vi "Get Fit Results String.vi"(7 "Plot Name":string, 8 "error in (no error)":errorcluster, 9 "Fit Parameters Uncertainties Cluster":variant, 10 "Fit Model":T1, 11 "Fit Parameters Cluster":variant) -> (0 "error out":errorcluster, 3 "Fit Results String":string)   [LabVIEW 2019]
uses:
  Fit Models.ctl
  Gaussian Fit Results v2.ctl
  Lorentzian Fit Results v2.ctl
  Asymmetric Gaussian Fit Results v2.ctl
  Asymmetric Lorentzian Fit Results v2.ctl
  Gaussian-Lorentzian Fit Results v2.ctl
  Lorentzian-Gaussian Fit Results v2.ctl
  Two H-Connected Gaussians Fit Parameters.ctl
  Two T-Connected Gaussians Fit Parameters.ctl
  Two T-Connected Asymmetric Gaussians Fit Parameters.ctl
  Two H-Connected Asymmetric Gaussians Fit Parameters.ctl
  Single Exponential Fit Parameters v2.ctl
  Double Exponential Fit Parameters v2.ctl
  2D Gaussian ACF Fit Results.ctl
  2D Gaussian + Blinking ACF Fit Results.ctl
  2D Gaussian + Flow ACF Fit Results.ctl
  3D Gaussian ACF Fit Results.ctl
  3D Gaussian + Blinking ACF Fit Results.ctl
  2D Gaussian ACF & 2D Gaussian ACF + Flow Fit Results.ctl
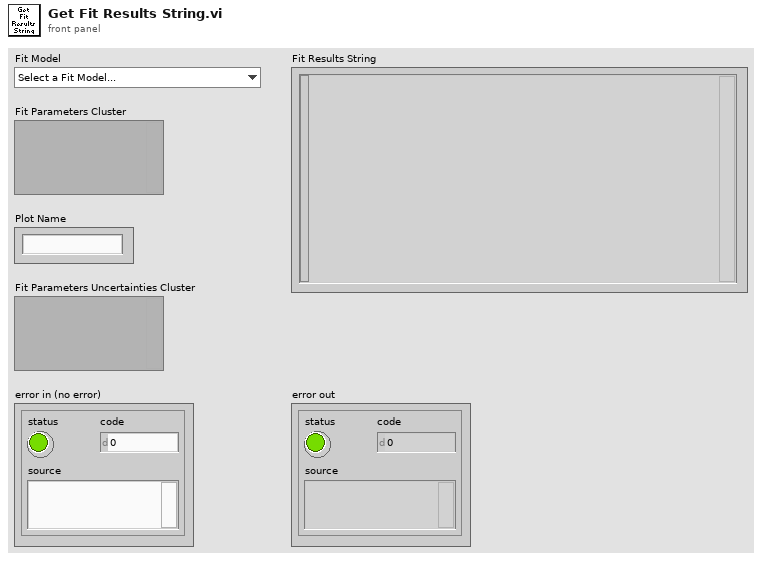
[diagram p1: front panel]
types:
  T1 = typedef "Fit Models.ctl" = enum16{"Select a Fit Model...", "           Single Peak", "Gaussian", "Asymmetric Gaussian", "Lorentzian", "Asymmetric Lorentzian", "Gaussian/Lorentzian", "Lorentzian/Gaussian", "           Double Peak", "Two Gaussians", "Two Asymmetric Gaussians", "Two H-Connected Gaussians", "Two T-Connected Gaussians", "Two H-Connected Asymmetric Gaussians", "Two T-Connected Asymmetric Gaussians", "           Triple Peak", "Three Gaussians", "Three Asymmetric Gaussians", "              Decays", "Single Exponential", "Two Exponentials", "               ACF", "2D Gaussian ACF", "2D Gaussian + Blinking ACF", "2D Gaussian + Flow ACF", "3D Gaussian ACF", "3D Gaussian + Blinking ACF", "             Multiplot", "2D Gaussian ACF & 2D Gaussian + Flow ACF"}
  T2 = typedef "Gaussian Fit Results v2.ctl" = cluster{"Amplitude":dbl, "Peak":dbl, "SDV":dbl, "FWHM":dbl, "Integral":dbl, "RMSE":dbl, "R^2":dbl}
  T3 = typedef "Lorentzian Fit Results v2.ctl" = cluster{"Amplitude":dbl, "Peak":dbl, "FWHM":dbl, "Integral":dbl, "RMSE":dbl, "R^2":dbl}
  T4 = typedef "Asymmetric Gaussian Fit Results v2.ctl" = cluster{"Amplitude":dbl, "Peak":dbl, "SDV-":dbl, "SDV+":dbl, "Mean":dbl, "SDV":dbl, "FWHM":dbl, "Integral":dbl, "RMSE":dbl, "R^2":dbl}
  T5 = typedef "Asymmetric Lorentzian Fit Results v2.ctl" = cluster{"Amplitude":dbl, "Peak":dbl, "FWHM-":dbl, "FWHM+":dbl, "Integral":dbl, "RMSE":dbl, "R^2":dbl}
  T6 = typedef "Gaussian-Lorentzian Fit Results v2.ctl" = cluster{"Amplitude":dbl, "Peak":dbl, "SDV-":dbl, "FWHM+":dbl, "Mean":dbl, "FWHM":dbl, "Integral":dbl, " RMSE":dbl, "R^2":dbl}
  T7 = typedef "Lorentzian-Gaussian Fit Results v2.ctl" = cluster{"Amplitude":dbl, "Peak":dbl, "FWHM-":dbl, "SDV+":dbl, "Mean":dbl, "FWHM":dbl, "Integral":dbl, "RMSE":dbl, "R^2":dbl}
  T8 = typedef "Two H-Connected Gaussians Fit Parameters.ctl" = cluster{"Gaussian Parameters":T2[], "Bridge Amplitude ":dbl}
  T9 = typedef "Two T-Connected Gaussians Fit Parameters.ctl" = cluster{"Gaussian Parameters":T2[], "Bridge Amplitude ":dbl, "Bridge Slope":dbl}
  T10 = typedef "Two T-Connected Asymmetric Gaussians Fit Parameters.ctl" = cluster{"Asymmetric Gaussian Parameters":T4[], "Bridge Amplitude":dbl, "Bridge Slope":dbl}
  T11 = typedef "Two H-Connected Asymmetric Gaussians Fit Parameters.ctl" = cluster{"Asymmetric Gaussian Parameters":T4[], "Bridge Amplitude":dbl}
  T12 = typedef "Single Exponential Fit Parameters v2.ctl" = cluster{"Amplitude":dbl, "Time Constant":dbl, "Mean":dbl, "SDV":dbl, "FWHM":dbl, "Integral":dbl, "MSE":dbl, "R^2":dbl}
  T13 = typedef "Double Exponential Fit Parameters v2.ctl" = cluster{"A1":dbl, "tau1":dbl, "A2":dbl, "tau2":dbl, "Mean":dbl, "SDV":dbl, "Integral":dbl, "MSE":dbl, "R^2":dbl}
  T14 = typedef "2D Gaussian ACF Fit Results.ctl" = cluster{"Amplitude":dbl, "Diffusion Time":dbl, "RMSE":dbl, "R^2":dbl}
  T15 = typedef "2D Gaussian + Blinking ACF Fit Results.ctl" = cluster{"Amplitude":dbl, "Diffusion Time":dbl, "Blinking Fraction":dbl, "Blinking Time Constant":dbl, "RMSE":dbl, "R^2":dbl}
  T16 = typedef "2D Gaussian + Flow ACF Fit Results.ctl" = cluster{"Amplitude":dbl, "Diffusion Time":dbl, "Translation Time":dbl, "RMSE":dbl, "R^2":dbl}
  T17 = typedef "3D Gaussian ACF Fit Results.ctl" = cluster{"Amplitude":dbl, "Diffusion Time":dbl, "Aspect Ratio":dbl, "RMSE":dbl, "R^2":dbl}
  T18 = typedef "3D Gaussian + Blinking ACF Fit Results.ctl" = cluster{"Amplitude":dbl, "Diffusion Time":dbl, "Aspect Ratio":dbl, "Blinking Fraction":dbl, "Blinking Time Constant":dbl, "RMSE":dbl, "R^2":dbl}
  T19 = typedef "2D Gaussian ACF & 2D Gaussian ACF + Flow Fit Results.ctl" = cluster{"Amplitude 1":dbl, "Diffusion Time":dbl, "Amplitude 2":dbl, "Translation Time":dbl, "RMSE":dbl, "R^2":dbl}
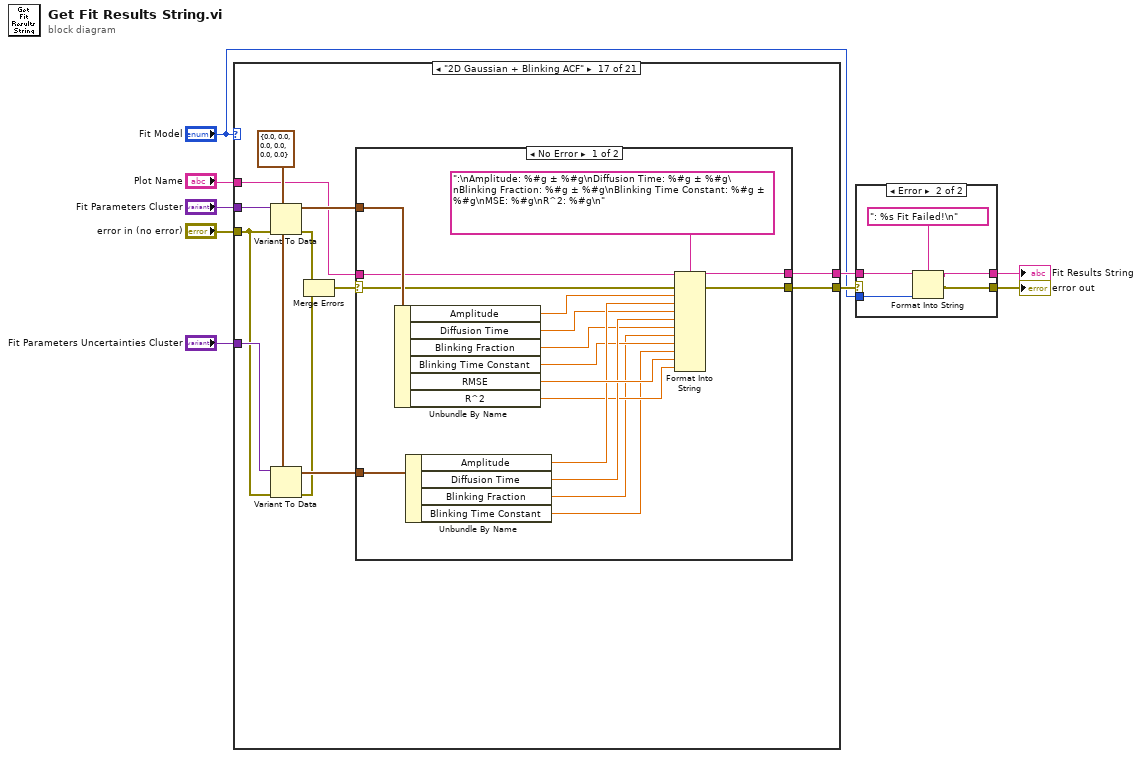
[diagram p0: block diagram]
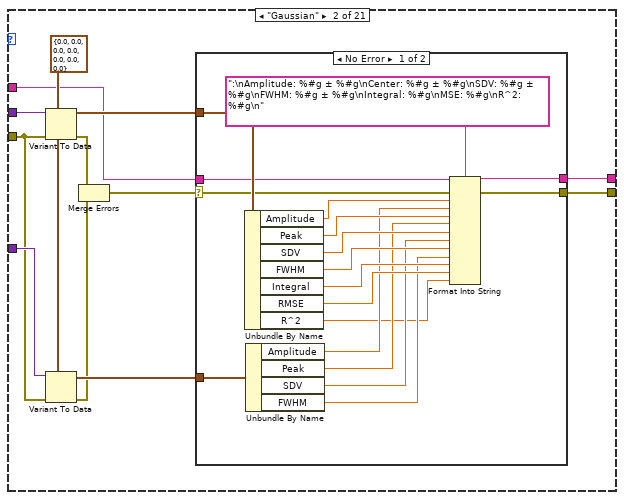
[diagram p4: hidden frame]
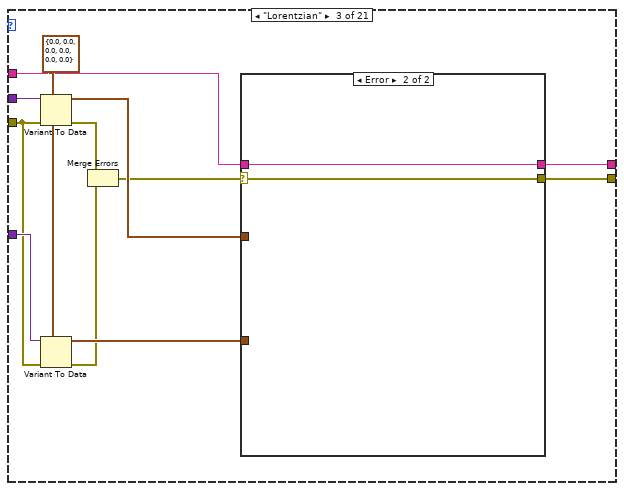
[diagram p6: hidden frame]
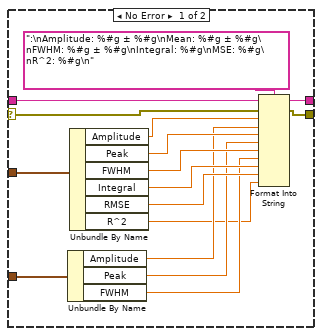
[diagram p7: hidden frame]
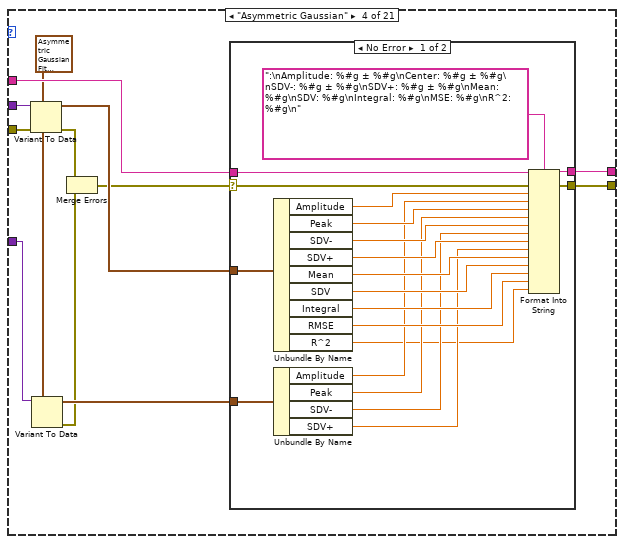
[diagram p8: hidden frame]
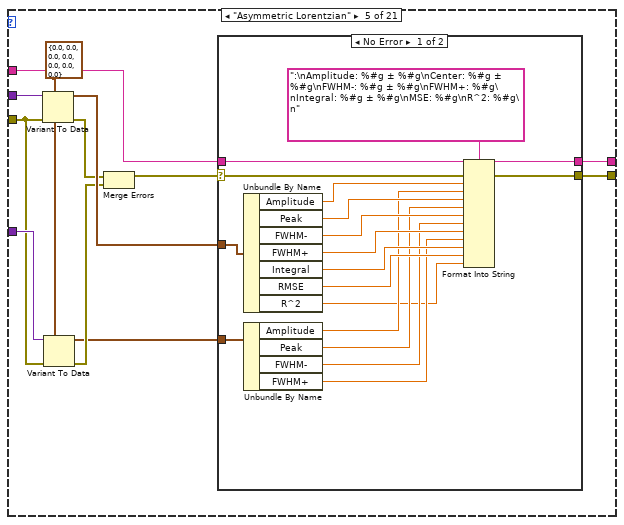
[diagram p10: hidden frame]
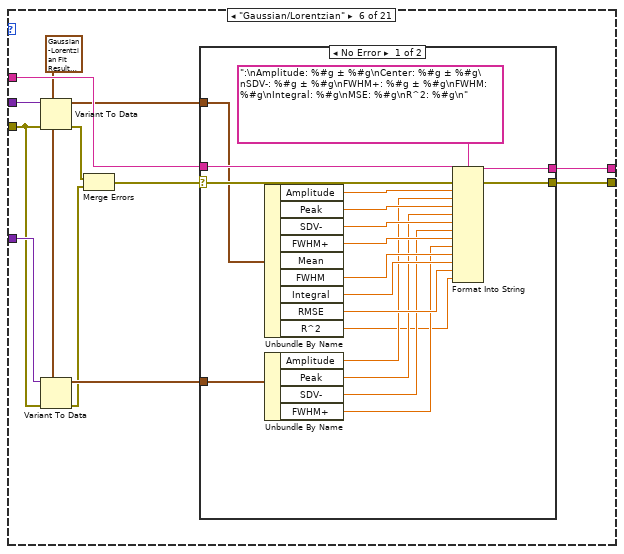
[diagram p12: hidden frame]
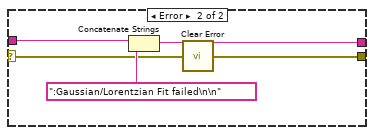
[diagram p13: hidden frame]
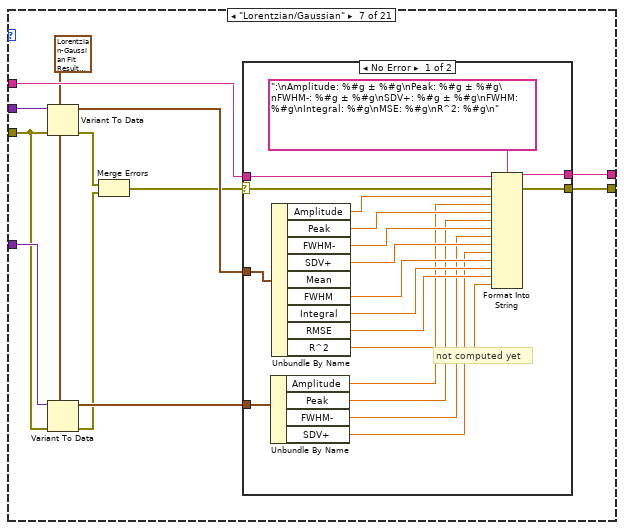
[diagram p14: hidden frame]
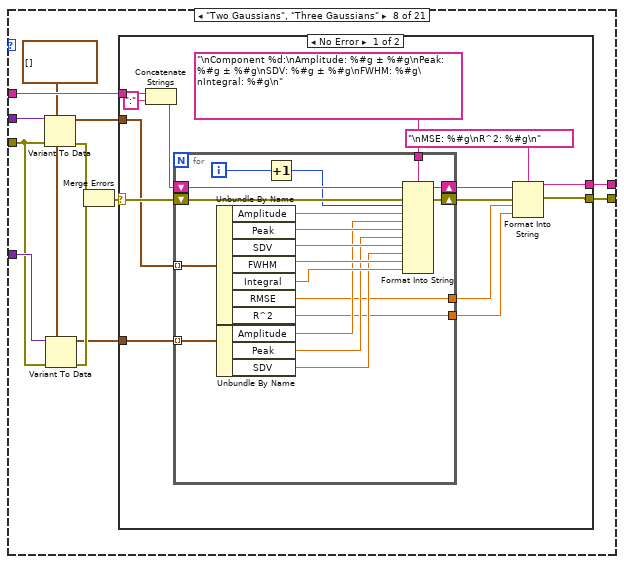
[diagram p16: hidden frame]
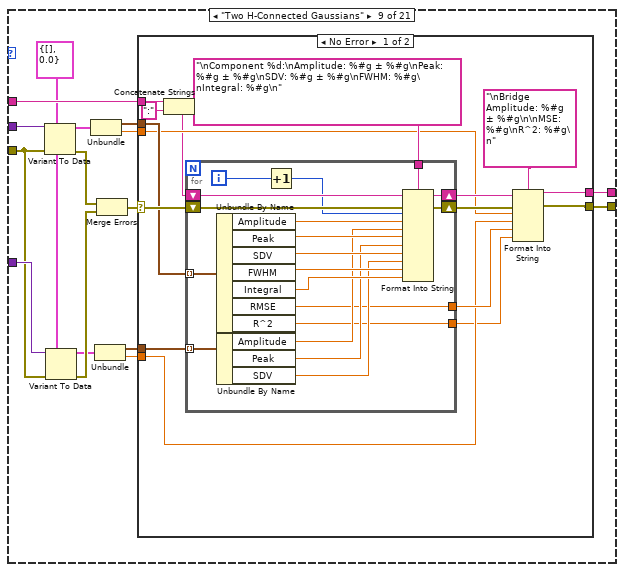
[diagram p18: hidden frame]
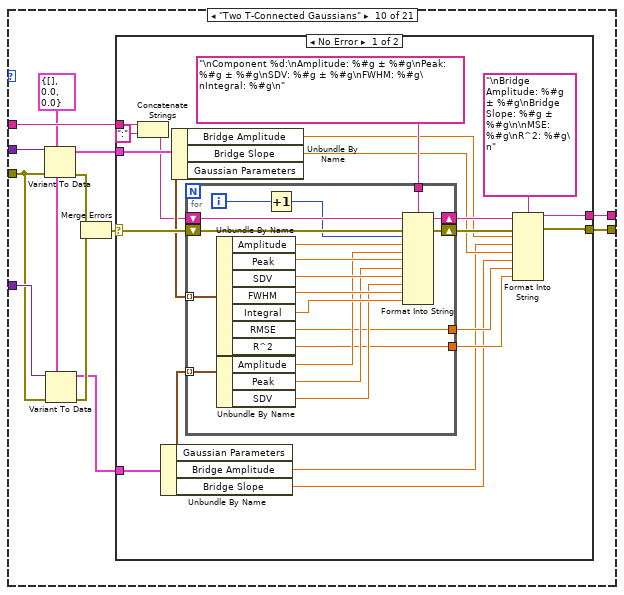
[diagram p20: hidden frame]
diagram:
  n1 = case shown="\"2D Gaussian + Blinking ACF\"" "Fit Model" {
    tunnel: "error in (no error)" -> [w10 w15 w46 w81 w110 w141 w175 w214 w265 w314 w366 w417 w474 w530 w561 w592 w619 w650 w679 w709 w742]
    tunnel: [w10 w22 w53 w83 w118 w149 w185 w218 w269 w318 w371 w422 w479 w533 w564 w599 w626 w657 w686 w715 w748] -> w5
    tunnel: [_ w21 w54 w84 w117 w150 w186 w219 w270 w319 w372 w423 w480 w534 w565 w598 w625 w656 w685 w714 w747] -> w3
    tunnel: "Fit Parameters Cluster" -> [_ w20 w52 w82 w115 w147 w183 w216 w267 w316 w369 w420 w477 w529 w563 w597 w624 w655 w684 w713 w746]
    tunnel: "Fit Parameters Uncertainties Cluster" -> [_ w18 w50 w76 w111 w142 w179 w215 w266 w315 w367 w418 w475 _ w562 w595 w622 w653 w682 w711 w744]
    tunnel: "Plot Name" -> [_ w11 w47 w80 w116 w148 w184 w217 w268 w317 w370 w421 w478 w524 w554 w588 w615 w646 w675 w705 w738]
    frame "Select a Fit Model...", Default {
    }
    frame "Gaussian" {
      w17 = T2 {"Amplitude"=0.0, "Peak"=0.0, "SDV"=0.0, "FWHM"=0.0, "Integral"=0.0, "RMSE"=0.0, "R^2"=0.0} ("Gaussian Fit Parameters")
      n2 = Variant To Data(error in=w15, type=w17, Variant=w20) -> (data=w19:T2, error out=w14:errorcluster)
      n3 = Variant To Data(error in=w15, type=w17, Variant=w18) -> (data=w16:T2, error out=w13:errorcluster)
      n4 = Merge Errors(w14, w13) -> (w12:errorcluster)
      n5 = case shown="No Error" w12 {
        selector: w12 -> [w30 w41]
        tunnel: [w40 w41] -> w22
        tunnel: [w39 w42] -> w21
        tunnel: w11 -> [w24 w42]
        tunnel: w19 -> [w37 _]
        tunnel: w16 -> [w29 _]
        frame No Error {
          n6 = Unbundle By Name(w37) -> ("Amplitude"=w36:dbl, "Peak"=w35:dbl, "SDV"=w34:dbl, "FWHM"=w32:dbl, "Integral"=w33:dbl, "RMSE"=w31:dbl, "R^2"=w23:dbl)
          n7 = Unbundle By Name(w29) -> ("Amplitude"=w28:dbl, "Peak"=w27:dbl, "SDV"=w26:dbl, "FWHM"=w25:dbl)
          n8 = Format Into String(format string=":\nAmplitude: %#g ± %#g\nCenter: %#g ± %#g\nSDV: %#g ± %#g\nFWHM: %#g ± %#g\nIntegral: %#g\nMSE: %#g\nR^2: %#g\n", initial string=w24, error in=w30, w36, w28, w35, w27, w34, w26, w32, w25, w33, w31, w23) -> (resulting string=w39:string, error out=w40:errorcluster)
        }
        frame Error {
        }
      }
    }
    frame "Lorentzian" {
      w48 = T3 {"Amplitude"=0.0, "Peak"=0.0, "FWHM"=0.0, "Integral"=0.0, "RMSE"=0.0, "R^2"=0.0} ("Lorentz Fit Parameters")
      n9 = Variant To Data(error in=w46, type=w48, Variant=w52) -> (data=w51:T3, error out=w45:errorcluster)
      n10 = Variant To Data(error in=w46, type=w48, Variant=w50) -> (data=w49:T3, error out=w44:errorcluster)
      n11 = Merge Errors(w45, w44) -> (w43:errorcluster)
      n12 = case shown="Error" w43 {
        selector: w43 -> [w61 w71]
        tunnel: w47 -> [w70 w72]
        tunnel: w51 -> [w69 _]
        tunnel: [w63 w72] -> w54
        tunnel: [w62 w71] -> w53
        tunnel: w49 -> [w59 _]
        frame No Error {
          n13 = Unbundle By Name(w59) -> ("Amplitude"=w58:dbl, "Peak"=w57:dbl, "FWHM"=w56:dbl)
          n14 = Unbundle By Name(w69) -> ("Amplitude"=w67:dbl, "Peak"=w68:dbl, "FWHM"=w66:dbl, "Integral"=w65:dbl, "RMSE"=w64:dbl, "R^2"=w55:dbl)
          n15 = Format Into String(format string=":\nAmplitude: %#g ± %#g\nMean: %#g ± %#g\nFWHM: %#g ± %#g\nIntegral: %#g\nMSE: %#g\nR^2: %#g\n", initial string=w70, error in=w61, w67, w58, w68, w57, w66, w56, w65, w64, w55) -> (resulting string=w63:string, error out=w62:errorcluster)
        }
        frame Error {
        }
      }
    }
    frame "Asymmetric Gaussian" {
      w78 = T4 {"Amplitude"=0.0, "Peak"=0.0, "SDV-"=0.0, "SDV+"=0.0, "Mean"=0.0, "SDV"=0.0, "FWHM"=0.0, "Integral"=0.0, "RMSE"=0.0, "R^2"=0.0} ("Asymmetric Gaussian Fit Parameters")
      n16 = Variant To Data(error in=w81, type=w78, Variant=w82) -> (data=w79:T4, error out=w75:errorcluster)
      n17 = Variant To Data(type=w78, Variant=w76) -> (data=w77:T4, error out=w74:errorcluster)  [unwired: 1 in]
      n18 = Merge Errors(w75, w74) -> (w73:errorcluster)
      n19 = case shown="No Error" w73 {
        selector: w73 -> [w102 w106]
        tunnel: w80 -> [w104 w105]
        tunnel: w79 -> [w91 _]
        tunnel: [w93 w105] -> w84
        tunnel: [w92 w106] -> w83
        tunnel: w77 -> [w90 _]
        frame No Error {
          n20 = Unbundle By Name(w91) -> ("Amplitude"=w98:dbl, "Peak"=w101:dbl, "SDV-"=w100:dbl, "SDV+"=w99:dbl, "Mean"=w97:dbl, "SDV"=w96:dbl, "Integral"=w95:dbl, "RMSE"=w94:dbl, "R^2"=w85:dbl)
          n21 = Unbundle By Name(w90) -> ("Amplitude"=w89:dbl, "Peak"=w88:dbl, "SDV-"=w87:dbl, "SDV+"=w86:dbl)
          n22 = Format Into String(format string=":\nAmplitude: %#g ± %#g\nCenter: %#g ± %#g\nSDV-: %#g ± %#g\nSDV+: %#g ± %#g\nMean: %#g\nSDV: %#g\nIntegral: %#g\nMSE: %#g\nR^2: %#g\n", initial string=w104, error in=w102, w98, w89, w101, w88, w100, w87, w99, w86, w97, w96, w95, w94, w85) -> (resulting string=w93:string, error out=w92:errorcluster)
        }
        frame Error {
        }
      }
    }
    frame "Asymmetric Lorentzian" {
      w112 = T5 {"Amplitude"=0.0, "Peak"=0.0, "FWHM-"=0.0, "FWHM+"=0.0, "Integral"=0.0, "RMSE"=0.0, "R^2"=0.0} ("Asymmetric Lorentz Fit Parameters")
      n23 = Variant To Data(error in=w110, type=w112, Variant=w115) -> (data=w114:T5, error out=w113:errorcluster)
      n24 = Variant To Data(error in=w110, type=w112, Variant=w111) -> (data=w108:T5, error out=w109:errorcluster)
      n25 = Merge Errors(w113, w109) -> (w107:errorcluster)
      n26 = case shown="No Error" w107 {
        selector: w107 -> [w135 w138]
        tunnel: [w128 w138] -> w118
        tunnel: [w127 w137] -> w117
        tunnel: w116 -> [w122 w137]
        tunnel: w114 -> [w121 _]
        tunnel: w108 -> [w120 _]
        frame No Error {
          n27 = Unbundle By Name(w121) -> ("Amplitude"=w131:dbl, "Peak"=w134:dbl, "FWHM-"=w133:dbl, "FWHM+"=w132:dbl, "Integral"=w130:dbl, "RMSE"=w129:dbl, "R^2"=w119:dbl)
          n28 = Unbundle By Name(w120) -> ("Amplitude"=w126:dbl, "Peak"=w125:dbl, "FWHM-"=w124:dbl, "FWHM+"=w123:dbl)
          n29 = Format Into String(format string=":\nAmplitude: %#g ± %#g\nCenter: %#g ± %#g\nFWHM-: %#g ± %#g\nFWHM+: %#g\nIntegral: %#g ± %#g\nMSE: %#g\nR^2: %#g\n", initial string=w122, error in=w135, w131, w126, w134, w125, w133, w124, w132, w123, w130, w129, w119) -> (resulting string=w127:string, error out=w128:errorcluster)
        }
        frame Error {
        }
      }
    }
    frame "Gaussian/Lorentzian" {
      w143 = T6 {"Amplitude"=0.0, "Peak"=0.0, "SDV-"=0.0, "FWHM+"=0.0, "Mean"=0.0, "FWHM"=0.0, "Integral"=0.0, " RMSE"=0.0, "R^2"=0.0} ("Gaussian/Lorentzian Fit Parameters")
      n30 = Variant To Data(error in=w141, type=w143, Variant=w147) -> (data=w144:T6, error out=w146:errorcluster)
      n31 = Variant To Data(error in=w141, type=w143, Variant=w142) -> (data=w140:T6, error out=w139:errorcluster)
      n32 = Merge Errors(w146, w139) -> (w145:errorcluster)
      n33 = case shown="No Error" w145 {
        selector: w145 -> [w167 w171]
        tunnel: w148 -> [w169 w173]
        tunnel: [w159 w172] -> w150
        tunnel: [w158 w170] -> w149
        tunnel: w144 -> [w153 _]
        tunnel: w140 -> [w152 _]
        frame No Error {
          n34 = Unbundle By Name(w153) -> ("Amplitude"=w165:dbl, "Peak"=w166:dbl, "SDV-"=w164:dbl, "FWHM+"=w163:dbl, "FWHM"=w162:dbl, "Integral"=w161:dbl, "RMSE"=w160:dbl, "R^2"=w151:dbl)  [unwired: 1 out]
          n35 = Unbundle By Name(w152) -> ("Amplitude"=w157:dbl, "Peak"=w156:dbl, "SDV-"=w155:dbl, "FWHM+"=w154:dbl)
          n36 = Format Into String(format string=":\nAmplitude: %#g ± %#g\nCenter: %#g ± %#g\nSDV-: %#g ± %#g\nFWHM+: %#g ± %#g\nFWHM: %#g\nIntegral: %#g\nMSE: %#g\nR^2: %#g\n", initial string=w169, error in=w167, w165, w157, w166, w156, w164, w155, w163, w154, w162, w161, w160, w151) -> (resulting string=w159:string, error out=w158:errorcluster)
        }
        frame Error {
          n37 = Concatenate Strings(w173, ":Gaussian/Lorentzian Fit failed\n\n" ("format string")) -> (w172:string)
          n38 = call "Clear Error.vi"("Error In"=w171) -> ("no Error Out"=w170:errorcluster)  [unwired: 8 in]
        }
      }
    }
    frame "Lorentzian/Gaussian" {
      w178 = T7 {"Amplitude"=0.0, "Peak"=0.0, "FWHM-"=0.0, "SDV+"=0.0, "Mean"=0.0, "FWHM"=0.0, "Integral"=0.0, "RMSE"=0.0, "R^2"=0.0} ("Lorentzian/Gaussian Fit Parameters")
      n39 = Variant To Data(error in=w175, type=w178, Variant=w183) -> (data=w182:T7, error out=w181:errorcluster)
      n40 = Variant To Data(error in=w175, type=w178, Variant=w179) -> (data=w177:T7, error out=w176:errorcluster)
      n41 = Merge Errors(w181, w176) -> (w180:errorcluster)
      n42 = case shown="No Error" w180 {
        selector: w180 -> [w204 w207]
        tunnel: [w196 w206] -> w186
        tunnel: [w195 w207] -> w185
        tunnel: w184 -> [w190 w206]
        tunnel: w182 -> [w189 _]
        tunnel: w177 -> [w188 _]
        frame No Error {
          # "not computed yet"
          n43 = Unbundle By Name(w188) -> ("Amplitude"=w194:dbl, "Peak"=w193:dbl, "FWHM-"=w192:dbl, "SDV+"=w191:dbl)
          n44 = Unbundle By Name(w189) -> ("Amplitude"=w202:dbl, "Peak"=w203:dbl, "FWHM-"=w200:dbl, "SDV+"=w201:dbl, "FWHM"=w199:dbl, "Integral"=w198:dbl, "RMSE"=w197:dbl, "R^2"=w187:dbl)  [unwired: 1 out]
          n45 = Format Into String(format string=":\nAmplitude: %#g ± %#g\nPeak: %#g ± %#g\nFWHM-: %#g ± %#g\nSDV+: %#g ± %#g\nFWHM: %#g\nIntegral: %#g\nMSE: %#g\nR^2: %#g\n", initial string=w190, error in=w204, w202, w194, w203, w193, w200, w192, w201, w191, w199, w198, w197, w187) -> (resulting string=w196:string, error out=w195:errorcluster)
        }
        frame Error {
        }
      }
    }
    frame "Two Gaussians", "Three Gaussians" {
      w208 = T2[] [] ("Array")
      n46 = Variant To Data(error in=w214, type=w208, Variant=w216) -> (data=w210:T2[], error out=w213:errorcluster)
      n47 = Variant To Data(error in=w214, type=w208, Variant=w215) -> (data=w209:T2[], error out=w212:errorcluster)
      n48 = Merge Errors(w213, w212) -> (w211:errorcluster)
      n49 = case shown="No Error" w211 {
        selector: w211 -> [w232 w254]
        tunnel: [w227 w253] -> w219
        tunnel: [w225 w254] -> w218
        tunnel: w217 -> [w230 w253]
        tunnel: w210 -> [w229 _]
        tunnel: w209 -> [w228 _]
        frame No Error {
          n50 = Concatenate Strings(w230, ":" ("string")) -> (w221:string)
          n51 = for {
            tunnel: "\nComponent %d:\nAmplitude: %#g ± %#g\nPeak: %#g ± %#g\nSDV: %#g ± %#g\nFWHM: %#g\nIntegral: %#g\n" ("format string") -> [w252]
            shift-right: [w245] -> w226
            shift-left: w232 -> [w251]
            shift-right: [w246] -> w231
            shift-left: w221 -> [w244]
            tunnel: w229 -> [w237] mode=indexing
            tunnel: w228 -> [w236] mode=indexing
            tunnel: [w235] -> w223
            tunnel: [w234] -> w222
            i -> [w239]
            n52 = Unbundle By Name(w237) -> ("Amplitude"=w240:dbl, "Peak"=w250:dbl, "SDV"=w249:dbl, "FWHM"=w248:dbl, "Integral"=w247:dbl, "RMSE"=w235:dbl, "R^2"=w234:dbl)
            n53 = Unbundle By Name(w236) -> ("Amplitude"=w243:dbl, "Peak"=w242:dbl, "SDV"=w241:dbl)
            n54 = Increment(x=w239) -> (x+1=w238:i32)
            n55 = Format Into String(format string=w252, initial string=w244, error in=w251, w238, w240, w243, w250, w242, w249, w241, w248, w247) -> (resulting string=w246:string, error out=w245:errorcluster)
          }
          n56 = Format Into String(format string="\nMSE: %#g\nR^2: %#g\n", initial string=w231, error in=w226, w223, w222) -> (resulting string=w227:string, error out=w225:errorcluster)
        }
        frame Error {
        }
      }
    }
    frame "Two H-Connected Gaussians" {
      w259 = T8 {"Gaussian Parameters"=[], "Bridge Amplitude "=0.0} ("Bridged Gaussians Parameters")
      n57 = Variant To Data(error in=w265, type=w259, Variant=w267) -> (data=w261:T8, error out=w264:errorcluster)
      n58 = Variant To Data(error in=w265, type=w259, Variant=w266) -> (data=w260:T8, error out=w263:errorcluster)
      n59 = Unbundle(w261) -> ("Gaussian Parameters"=w258:T2[], "Bridge Amplitude"=w256:dbl)
      n60 = Unbundle(w260) -> ("Gaussian Parameters"=w257:T2[], "Bridge Amplitude"=w255:dbl)
      n61 = Merge Errors(w264, w263) -> (w262:errorcluster)
      n62 = case shown="No Error" w262 {
        selector: w262 -> [w285 w307]
        tunnel: [w281 w306] -> w270
        tunnel: [w279 w307] -> w269
        tunnel: w268 -> [w272 w306]
        tunnel: w258 -> [w283 _]
        tunnel: w257 -> [w282 _]
        tunnel: w256 -> [w275 _]
        tunnel: w255 -> [w276 _]
        frame No Error {
          n63 = Concatenate Strings(w272, ":" ("string")) -> (w271:string)
          n64 = for {
            tunnel: "\nComponent %d:\nAmplitude: %#g ± %#g\nPeak: %#g ± %#g\nSDV: %#g ± %#g\nFWHM: %#g\nIntegral: %#g\n" ("format string") -> [w305]
            shift-right: [w298] -> w280
            shift-left: w285 -> [w304]
            shift-right: [w299] -> w284
            shift-left: w271 -> [w297]
            tunnel: w283 -> [w290] mode=indexing
            tunnel: w282 -> [w289] mode=indexing
            tunnel: [w288] -> w277
            tunnel: [w287] -> w274
            i -> [w292]
            n65 = Unbundle By Name(w290) -> ("Amplitude"=w293:dbl, "Peak"=w303:dbl, "SDV"=w302:dbl, "FWHM"=w301:dbl, "Integral"=w300:dbl, "RMSE"=w288:dbl, "R^2"=w287:dbl)
            n66 = Unbundle By Name(w289) -> ("Amplitude"=w296:dbl, "Peak"=w295:dbl, "SDV"=w294:dbl)
            n67 = Increment(x=w292) -> (x+1=w291:i32)
            n68 = Format Into String(format string=w305, initial string=w297, error in=w304, w291, w293, w296, w303, w295, w302, w294, w301, w300) -> (resulting string=w299:string, error out=w298:errorcluster)
          }
          n69 = Format Into String(format string="\nBridge Amplitude: %#g ± %#g\n\nMSE: %#g\nR^2: %#g\n", initial string=w284, error in=w280, w275, w276, w277, w274) -> (resulting string=w281:string, error out=w279:errorcluster)
        }
        frame Error {
        }
      }
    }
    frame "Two T-Connected Gaussians" {
      w310 = T9 {"Gaussian Parameters"=[], "Bridge Amplitude "=0.0, "Bridge Slope"=0.0} ("Bridged Gaussians Parameters")
      n70 = Variant To Data(error in=w314, type=w310, Variant=w316) -> (data=w309:T9, error out=w313:errorcluster)
      n71 = Variant To Data(error in=w314, type=w310, Variant=w315) -> (data=w308:T9, error out=w312:errorcluster)
      n72 = Merge Errors(w313, w312) -> (w311:errorcluster)
      n73 = case shown="No Error" w311 {
        selector: w311 -> [w338 w360]
        tunnel: [w336 w359] -> w319
        tunnel: [w334 w360] -> w318
        tunnel: w317 -> [w321 w359]
        tunnel: w309 -> [w330 _]
        tunnel: w308 -> [w326 _]
        frame No Error {
          n74 = Concatenate Strings(w321, ":" ("string")) -> (w320:string)
          n75 = Unbundle By Name(w326) -> ("Gaussian Parameters"=w325:T2[], "Bridge Amplitude"=w324:dbl, "Bridge Slope"=w323:dbl)
          n76 = Unbundle By Name(w330) -> ("Bridge Amplitude"=w328:dbl, "Bridge Slope"=w327:dbl, "Gaussian Parameters"=w329:T2[])
          n77 = for {
            tunnel: "\nComponent %d:\nAmplitude: %#g ± %#g\nPeak: %#g ± %#g\nSDV: %#g ± %#g\nFWHM: %#g\nIntegral: %#g\n" ("format string") -> [w358]
            shift-right: [w351] -> w335
            shift-left: w338 -> [w357]
            shift-right: [w352] -> w337
            shift-left: w320 -> [w350]
            tunnel: w329 -> [w343] mode=indexing
            tunnel: w325 -> [w342] mode=indexing
            tunnel: [w341] -> w332
            tunnel: [w340] -> w331
            i -> [w345]
            n78 = Unbundle By Name(w343) -> ("Amplitude"=w346:dbl, "Peak"=w356:dbl, "SDV"=w355:dbl, "FWHM"=w354:dbl, "Integral"=w353:dbl, "RMSE"=w341:dbl, "R^2"=w340:dbl)
            n79 = Unbundle By Name(w342) -> ("Amplitude"=w349:dbl, "Peak"=w348:dbl, "SDV"=w347:dbl)
            n80 = Increment(x=w345) -> (x+1=w344:i32)
            n81 = Format Into String(format string=w358, initial string=w350, error in=w357, w344, w346, w349, w356, w348, w355, w347, w354, w353) -> (resulting string=w352:string, error out=w351:errorcluster)
          }
          n82 = Format Into String(format string="\nBridge Amplitude: %#g ± %#g\nBridge Slope: %#g ± %#g\n\nMSE: %#g\nR^2: %#g\n", initial string=w337, error in=w335, w328, w324, w327, w323, w332, w331) -> (resulting string=w336:string, error out=w334:errorcluster)
        }
        frame Error {
        }
      }
    }
    frame "Two Asymmetric Gaussians", "Three Asymmetric Gaussians" {
      w365 = T4[] [] ("Array")
      n83 = Variant To Data(error in=w366, type=w365, Variant=w367) -> (data=w361:T4[], error out=w364:errorcluster)
      n84 = Variant To Data(error in=w366, type=w365, Variant=w369) -> (data=w362:T4[], error out=w368:errorcluster)
      n85 = Merge Errors(w368, w364) -> (w363:errorcluster)
      n86 = case shown="No Error" w363 {
        selector: w363 -> [w385 w410]
        tunnel: w370 -> [w386 w411]
        tunnel: [w378 w411] -> w372
        tunnel: [w376 w410] -> w371
        tunnel: w362 -> [w384 _]
        tunnel: w361 -> [w383 _]
        frame No Error {
          n87 = Concatenate Strings(w386, ":" ("string")) -> (w381:string)
          n88 = for {
            shift-right: [w399] -> w379
            shift-left: w381 -> [w402]
            shift-right: [w400] -> w377
            shift-left: w385 -> [w401]
            tunnel: w384 -> [w398] mode=indexing
            tunnel: w383 -> [w397] mode=indexing
            tunnel: "\nComponent %d:\nAmplitude: %#g ± %#g\nCenter: %#g ± %#g\nSDV-: %#g ± %#g\nSDV+: %#g ± %#g\nMean: %#g\nSDV: %#g\nFWHM: %#g\nIntegral: %#g\n" ("format string") -> [w396]
            tunnel: [w388] -> w375
            tunnel: [w387] -> w373
            i -> [w394]
            n89 = Unbundle By Name(w398) -> ("Amplitude"=w395:dbl, "Peak"=w409:dbl, "SDV-"=w408:dbl, "SDV+"=w407:dbl, "Mean"=w406:dbl, "SDV"=w405:dbl, "FWHM"=w404:dbl, "Integral"=w403:dbl, "RMSE"=w388:dbl, "R^2"=w387:dbl)
            n90 = Unbundle By Name(w397) -> ("Amplitude"=w392:dbl, "Peak"=w391:dbl, "SDV-"=w390:dbl, "SDV+"=w389:dbl)
            n91 = Increment(x=w394) -> (x+1=w393:i32)
            n92 = Format Into String(format string=w396, initial string=w402, error in=w401, w393, w395, w392, w409, w391, w408, w390, w407, w389, w406, w405, w404, w403) -> (resulting string=w399:string, error out=w400:errorcluster)
          }
          n93 = Format Into String(format string="\nMSE: %#g\nR^2: %#g\n", initial string=w379, error in=w377, w375, w373) -> (resulting string=w378:string, error out=w376:errorcluster)
        }
        frame Error {
        }
      }
    }
    frame "Two T-Connected Asymmetric Gaussians" {
      w412 = T10 {"Asymmetric Gaussian Parameters"=[], "Bridge Amplitude"=0.0, "Bridge Slope"=0.0} ("Two T-Connected Asymmetric Gaussian Parameters")
      n94 = Variant To Data(error in=w417, type=w412, Variant=w418) -> (data=w413:T10, error out=w416:errorcluster)
      n95 = Variant To Data(error in=w417, type=w412, Variant=w420) -> (data=w414:T10, error out=w419:errorcluster)
      n96 = Merge Errors(w419, w416) -> (w415:errorcluster)
      n97 = case shown="No Error" w415 {
        selector: w415 -> [w442 w467]
        tunnel: w421 -> [w443 w468]
        tunnel: [w436 w468] -> w423
        tunnel: [w435 w467] -> w422
        tunnel: w414 -> [w441 _]
        tunnel: w413 -> [w427 _]
        frame No Error {
          n98 = Unbundle By Name(w441) -> ("Bridge Amplitude"=w431:dbl, "Bridge Slope"=w430:dbl, "Asymmetric Gaussian Parameters"=w428:T4[])
          n99 = Concatenate Strings(w443, ":" ("string")) -> (w439:string)
          n100 = Unbundle By Name(w427) -> ("Asymmetric Gaussian Parameters"=w426:T4[], "Bridge Amplitude"=w425:dbl, "Bridge Slope"=w424:dbl)
          n101 = for {
            shift-right: [w456] -> w437
            shift-left: w439 -> [w459]
            shift-right: [w457] -> w434
            shift-left: w442 -> [w458]
            tunnel: w428 -> [w455] mode=indexing
            tunnel: w426 -> [w454] mode=indexing
            tunnel: "\nComponent %d:\nAmplitude: %#g ± %#g\nCenter: %#g ± %#g\nSDV-: %#g ± %#g\nSDV+: %#g ± %#g\nMean: %#g\nSDV: %#g\nFWHM: %#g\nIntegral: %#g\n" ("format string") -> [w453]
            tunnel: [w445] -> w432
            tunnel: [w444] -> w429
            i -> [w451]
            n102 = Unbundle By Name(w455) -> ("Amplitude"=w452:dbl, "Peak"=w466:dbl, "SDV-"=w465:dbl, "SDV+"=w464:dbl, "Mean"=w463:dbl, "SDV"=w462:dbl, "FWHM"=w461:dbl, "Integral"=w460:dbl, "RMSE"=w445:dbl, "R^2"=w444:dbl)
            n103 = Unbundle By Name(w454) -> ("Amplitude"=w449:dbl, "Peak"=w448:dbl, "SDV-"=w447:dbl, "SDV+"=w446:dbl)
            n104 = Increment(x=w451) -> (x+1=w450:i32)
            n105 = Format Into String(format string=w453, initial string=w459, error in=w458, w450, w452, w449, w466, w448, w465, w447, w464, w446, w463, w462, w461, w460) -> (resulting string=w456:string, error out=w457:errorcluster)
          }
          n106 = Format Into String(format string="\nBridge Amplitude: %#g ± %#g\nBridge Slope: %#g ± %#g\n\nMSE: %#g\nR^2: %#g\n", initial string=w437, error in=w434, w431, w425, w430, w424, w432, w429) -> (resulting string=w436:string, error out=w435:errorcluster)
        }
        frame Error {
        }
      }
    }
    frame "Two H-Connected Asymmetric Gaussians" {
      w471 = T11 {"Asymmetric Gaussian Parameters"=[], "Bridge Amplitude"=0.0} ("output cluster")
      n107 = Variant To Data(error in=w474, type=w471, Variant=w475) -> (data=w469:T11, error out=w473:errorcluster)
      n108 = Variant To Data(error in=w474, type=w471, Variant=w477) -> (data=w470:T11, error out=w476:errorcluster)
      n109 = Merge Errors(w476, w473) -> (w472:errorcluster)
      n110 = case shown="No Error" w472 {
        selector: w472 -> [w497 w522]
        tunnel: w478 -> [w498 w523]
        tunnel: [w492 w523] -> w480
        tunnel: [w490 w522] -> w479
        tunnel: w470 -> [w485 _]
        tunnel: w469 -> [w484 _]
        frame No Error {
          n111 = Unbundle(w484) -> ("Asymmetric Gaussian Parameters"=w483:T4[], "Bridge Amplitude"=w482:dbl)
          n112 = Unbundle(w485) -> ("Asymmetric Gaussian Parameters"=w487:T4[], "Bridge Amplitude"=w486:dbl)
          n113 = Concatenate Strings(w498, ":" ("string")) -> (w495:string)
          n114 = for {
            shift-right: [w511] -> w493
            shift-left: w495 -> [w514]
            shift-right: [w512] -> w491
            shift-left: w497 -> [w513]
            tunnel: w487 -> [w510] mode=indexing
            tunnel: w483 -> [w509] mode=indexing
            tunnel: "\nComponent %d:\nAmplitude: %#g ± %#g\nCenter: %#g ± %#g\nSDV-: %#g ± %#g\nSDV+: %#g ± %#g\nMean: %#g\nSDV: %#g\nFWHM: %#g\nIntegral: %#g\n" ("format string") -> [w508]
            tunnel: [w500] -> w488
            tunnel: [w499] -> w481
            i -> [w506]
            n115 = Unbundle By Name(w510) -> ("Amplitude"=w507:dbl, "Peak"=w521:dbl, "SDV-"=w520:dbl, "SDV+"=w519:dbl, "Mean"=w518:dbl, "SDV"=w517:dbl, "FWHM"=w516:dbl, "Integral"=w515:dbl, "RMSE"=w500:dbl, "R^2"=w499:dbl)
            n116 = Unbundle By Name(w509) -> ("Amplitude"=w504:dbl, "Peak"=w503:dbl, "SDV-"=w502:dbl, "SDV+"=w501:dbl)
            n117 = Increment(x=w506) -> (x+1=w505:i32)
            n118 = Format Into String(format string=w508, initial string=w514, error in=w513, w505, w507, w504, w521, w503, w520, w502, w519, w501, w518, w517, w516, w515) -> (resulting string=w511:string, error out=w512:errorcluster)
          }
          n119 = Format Into String(format string="\nBridge Amplitude: %#g ± %#g\n\nMSE: %#g\nR^2: %#g\n", initial string=w493, error in=w491, w486, w482, w488, w481) -> (resulting string=w492:string, error out=w490:errorcluster)
        }
        frame Error {
        }
      }
    }
    frame "Single Exponential" {
      w531 = T12 {"Amplitude"=0.0, "Time Constant"=0.0, "Mean"=0.0, "SDV"=0.0, "FWHM"=0.0, "Integral"=0.0, "MSE"=0.0, "R^2"=0.0} ("Single Exponential Fit Parameters")
      n120 = Variant To Data(error in=w530, type=w531, Variant=w529) -> (data=w532:T12, error out=w527:errorcluster)
      n121 = Variant To Data(error in=w530, type=w531, Variant=w529) -> (data=w528:T12, error out=w526:errorcluster)
      n122 = Merge Errors(w527, w526) -> (w525:errorcluster)
      n123 = case shown="No Error" w525 {
        selector: w525 -> [w550 w553]
        tunnel: [w542 w552] -> w534
        tunnel: [w541 w553] -> w533
        tunnel: w532 -> [w538 _]
        tunnel: w528 -> [w537 _]
        tunnel: w524 -> [w536 w552]
        frame No Error {
          n124 = Unbundle By Name(w538) -> ("Amplitude"=w548:dbl, "Time Constant"=w549:dbl, "Mean"=w547:dbl, "SDV"=w546:dbl, "FWHM"=w545:dbl, "Integral"=w544:dbl, "MSE"=w543:dbl, "R^2"=w535:dbl)
          n125 = Unbundle By Name(w537) -> ("Amplitude"=w540:dbl, "Time Constant"=w539:dbl)
          n126 = Format Into String(format string=":\nAmplitude: %#g ± %#g\nTime Constant: %#g ± %#g\nMean: %#g\nSDV: %#g\nFWHM: %#g\nIntegral: %#g\nMSE: %#g\nR^2: %#g\n", initial string=w536, error in=w550, w548, w540, w549, w539, w547, w546, w545, w544, w543, w535) -> (resulting string=w542:string, error out=w541:errorcluster)
        }
        frame Error {
        }
      }
    }
    frame "Two Exponentials" {
      w558 = T13 {"A1"=0.0, "tau1"=0.0, "A2"=0.0, "tau2"=0.0, "Mean"=0.0, "SDV"=0.0, "Integral"=0.0, "MSE"=0.0, "R^2"=0.0} ("Double Exponential Fit Parameters")
      n127 = Variant To Data(error in=w561, type=w558, Variant=w563) -> (data=w560:T13, error out=w557:errorcluster)
      n128 = Variant To Data(error in=w561, type=w558, Variant=w562) -> (data=w559:T13, error out=w556:errorcluster)
      n129 = Merge Errors(w557, w556) -> (w555:errorcluster)
      n130 = case shown="No Error" w555 {
        selector: w555 -> [w584 w587]
        tunnel: [w575 w586] -> w565
        tunnel: [w574 w587] -> w564
        tunnel: w560 -> [w569 _]
        tunnel: w559 -> [w568 _]
        tunnel: w554 -> [w567 w586]
        frame No Error {
          n131 = Unbundle By Name(w568) -> ("A1"=w573:dbl, "tau1"=w572:dbl, "A2"=w571:dbl, "tau2"=w570:dbl)
          n132 = Unbundle By Name(w569) -> ("A1"=w582:dbl, "tau1"=w583:dbl, "A2"=w577:dbl, "tau2"=w576:dbl, "Mean"=w581:dbl, "SDV"=w580:dbl, "Integral"=w579:dbl, "MSE"=w578:dbl, "R^2"=w566:dbl)
          n133 = Format Into String(format string=":\nA1: %#g ± %#g\nTau 1: %#g ± %#g\nA2: %#g ± %#g\nTau 2: %#g ± %#g\nMean: %#g\nSDV: %#g\nIntegral: %#g\nMSE: %#g\nR^2: %#g\n", initial string=w567, error in=w584, w582, w573, w583, w572, w577, w571, w576, w570, w581, w580, w579, w578, w566) -> (resulting string=w575:string, error out=w574:errorcluster)
        }
        frame Error {
        }
      }
    }
    frame "2D Gaussian ACF" {
      w594 = T14 {"Amplitude"=0.0, "Diffusion Time"=0.0, "RMSE"=0.0, "R^2"=0.0} ("2D ACF Fit Parameters")
      n134 = Variant To Data(error in=w592, type=w594, Variant=w597) -> (data=w596:T14, error out=w591:errorcluster)
      n135 = Variant To Data(error in=w592, type=w594, Variant=w595) -> (data=w593:T14, error out=w590:errorcluster)
      n136 = Merge Errors(w591, w590) -> (w589:errorcluster)
      n137 = case shown="No Error" w589 {
        selector: w589 -> [w606 w613]
        tunnel: [w612 w613] -> w599
        tunnel: [w611 w614] -> w598
        tunnel: w588 -> [w602 w614]
        tunnel: w596 -> [w609 _]
        tunnel: w593 -> [w605 _]
        frame No Error {
          n138 = Unbundle By Name(w609) -> ("Amplitude"=w608:dbl, "Diffusion Time"=w600:dbl, "RMSE"=w607:dbl, "R^2"=w601:dbl)
          n139 = Unbundle By Name(w605) -> ("Amplitude"=w604:dbl, "Diffusion Time"=w603:dbl)
          n140 = Format Into String(format string=":\nAmplitude: %#g ± %#g\nDiffusion Time: %#g ± %#g\nMSE: %#g\nR^2: %#g\n", initial string=w602, error in=w606, w608, w604, w600, w603, w607, w601) -> (resulting string=w611:string, error out=w612:errorcluster)
        }
        frame Error {
        }
      }
    }
    frame "2D Gaussian + Blinking ACF" {
      w621 = T15 {"Amplitude"=0.0, "Diffusion Time"=0.0, "Blinking Fraction"=0.0, "Blinking Time Constant"=0.0, "RMSE"=0.0, "R^2"=0.0} ("2D Gaussian + Blinking ACF Fit Parameters")
      n141 = Variant To Data(error in=w619, type=w621, Variant=w624) -> (data=w623:T15, error out=w618:errorcluster)
      n142 = Variant To Data(error in=w619, type=w621, Variant=w622) -> (data=w620:T15, error out=w617:errorcluster)
      n143 = Merge Errors(w618, w617) -> (w616:errorcluster)
      n144 = case shown="No Error" w616 {
        selector: w616 -> [w637 w644]
        tunnel: [w643 w644] -> w626
        tunnel: [w642 w645] -> w625
        tunnel: w615 -> [w633 w645]
        tunnel: w623 -> [w640 _]
        tunnel: w620 -> [w636 _]
        frame No Error {
          n145 = Unbundle By Name(w640) -> ("Amplitude"=w639:dbl, "Diffusion Time"=w631:dbl, "Blinking Fraction"=w630:dbl, "Blinking Time Constant"=w629:dbl, "RMSE"=w638:dbl, "R^2"=w632:dbl)
          n146 = Unbundle By Name(w636) -> ("Amplitude"=w635:dbl, "Diffusion Time"=w634:dbl, "Blinking Fraction"=w628:dbl, "Blinking Time Constant"=w627:dbl)
          n147 = Format Into String(format string=":\nAmplitude: %#g ± %#g\nDiffusion Time: %#g ± %#g\nBlinking Fraction: %#g ± %#g\nBlinking Time Constant: %#g ± %#g\nMSE: %#g\nR^2: %#g\n", initial string=w633, error in=w637, w639, w635, w631, w634, w630, w628, w629, w627, w638, w632) -> (resulting string=w642:string, error out=w643:errorcluster)
        }
        frame Error {
        }
      }
    }
    frame "2D Gaussian + Flow ACF" {
      w652 = T16 {"Amplitude"=0.0, "Diffusion Time"=0.0, "Translation Time"=0.0, "RMSE"=0.0, "R^2"=0.0} ("2D Gaussian + Blinking ACF Fit Parameters")
      n148 = Variant To Data(error in=w650, type=w652, Variant=w655) -> (data=w654:T16, error out=w649:errorcluster)
      n149 = Variant To Data(error in=w650, type=w652, Variant=w653) -> (data=w651:T16, error out=w648:errorcluster)
      n150 = Merge Errors(w649, w648) -> (w647:errorcluster)
      n151 = case shown="No Error" w647 {
        selector: w647 -> [w666 w673]
        tunnel: [w672 w673] -> w657
        tunnel: [w671 w674] -> w656
        tunnel: w646 -> [w662 w674]
        tunnel: w654 -> [w669 _]
        tunnel: w651 -> [w665 _]
        frame No Error {
          n152 = Unbundle By Name(w669) -> ("Amplitude"=w668:dbl, "Diffusion Time"=w660:dbl, "Translation Time"=w659:dbl, "RMSE"=w667:dbl, "R^2"=w661:dbl)
          n153 = Unbundle By Name(w665) -> ("Amplitude"=w664:dbl, "Diffusion Time"=w663:dbl, "Translation Time"=w658:dbl)
          n154 = Format Into String(format string=":\nAmplitude: %#g ± %#g\nDiffusion Time: %#g ± %#g\nTranslation Time Constant: %#g ± %#g\nMSE: %#g\nR^2: %#g\n", initial string=w662, error in=w666, w668, w664, w660, w663, w659, w658, w667, w661) -> (resulting string=w671:string, error out=w672:errorcluster)
        }
        frame Error {
        }
      }
    }
    frame "3D Gaussian ACF" {
      w681 = T17 {"Amplitude"=0.0, "Diffusion Time"=0.0, "Aspect Ratio"=0.0, "RMSE"=0.0, "R^2"=0.0} ("3D ACF Fit Parameters")
      n155 = Variant To Data(error in=w679, type=w681, Variant=w684) -> (data=w683:T17, error out=w678:errorcluster)
      n156 = Variant To Data(error in=w679, type=w681, Variant=w682) -> (data=w680:T17, error out=w677:errorcluster)
      n157 = Merge Errors(w678, w677) -> (w676:errorcluster)
      n158 = case shown="No Error" w676 {
        selector: w676 -> [w695 w702]
        tunnel: [w701 w702] -> w686
        tunnel: [w700 w703] -> w685
        tunnel: w675 -> [w692 w703]
        tunnel: w683 -> [w698 _]
        tunnel: w680 -> [w694 _]
        frame No Error {
          n159 = Unbundle By Name(w698) -> ("Amplitude"=w697:dbl, "Diffusion Time"=w690:dbl, "Aspect Ratio"=w688:dbl, "RMSE"=w696:dbl, "R^2"=w691:dbl)
          n160 = Unbundle By Name(w694) -> ("Amplitude"=w693:dbl, "Diffusion Time"=w689:dbl, "Aspect Ratio"=w687:dbl)
          n161 = Format Into String(format string=":\nAmplitude: %#g ± %#g\nDiffusion Time: %#g ± %#g\nAspect Ratio: %#g ± %#g\nMSE: %#g\nR^2: %#g\n", initial string=w692, error in=w695, w697, w693, w690, w689, w688, w687, w696, w691) -> (resulting string=w700:string, error out=w701:errorcluster)
        }
        frame Error {
        }
      }
    }
    frame "3D Gaussian + Blinking ACF" {
      w704 = T18 {"Amplitude"=0.0, "Diffusion Time"=0.0, "Aspect Ratio"=0.0, "Blinking Fraction"=0.0, "Blinking Time Constant"=0.0, "RMSE"=0.0, "R^2"=0.0} ("2D Gaussian + Blinking ACF Fit Parameters")
      n162 = Variant To Data(error in=w709, type=w704, Variant=w713) -> (data=w712:T18, error out=w708:errorcluster)
      n163 = Variant To Data(error in=w709, type=w704, Variant=w711) -> (data=w710:T18, error out=w707:errorcluster)
      n164 = Merge Errors(w708, w707) -> (w706:errorcluster)
      n165 = case shown="No Error" w706 {
        selector: w706 -> [w728 w735]
        tunnel: [w734 w735] -> w715
        tunnel: [w733 w736] -> w714
        tunnel: w705 -> [w724 w736]
        tunnel: w712 -> [w731 _]
        tunnel: w710 -> [w727 _]
        frame No Error {
          n166 = Unbundle By Name(w731) -> ("Amplitude"=w730:dbl, "Diffusion Time"=w722:dbl, "Aspect Ratio"=w717:dbl, "Blinking Fraction"=w721:dbl, "Blinking Time Constant"=w720:dbl, "RMSE"=w729:dbl, "R^2"=w723:dbl)
          n167 = Unbundle By Name(w727) -> ("Amplitude"=w726:dbl, "Diffusion Time"=w725:dbl, "Aspect Ratio"=w716:dbl, "Blinking Fraction"=w719:dbl, "Blinking Time Constant"=w718:dbl)
          n168 = Format Into String(format string=":\nAmplitude: %#g ± %#g\nDiffusion Time: %#g ± %#g\nAspect Ratio: %#g ± %#g\nBlinking Fraction: %#g ± %#g\nBlinking Time Constant: %#g ± %#g\nMSE: %#g\nR^2: %#g\n", initial string=w724, error in=w728, w730, w726, w722, w725, w717, w716, w721, w719, w720, w718, w729, w723) -> (resulting string=w733:string, error out=w734:errorcluster)
        }
        frame Error {
        }
      }
    }
    frame "2D Gaussian ACF & 2D Gaussian + Flow ACF" {
      w737 = T19 {"Amplitude 1"=0.0, "Diffusion Time"=0.0, "Amplitude 2"=0.0, "Translation Time"=0.0, "RMSE"=0.0, "R^2"=0.0} ("2D Gaussian ACF & ACF + Flow Fit Parameters")
      n169 = Variant To Data(error in=w742, type=w737, Variant=w746) -> (data=w745:T19, error out=w741:errorcluster)
      n170 = Variant To Data(error in=w742, type=w737, Variant=w744) -> (data=w743:T19, error out=w740:errorcluster)
      n171 = Merge Errors(w741, w740) -> (w739:errorcluster)
      n172 = case shown="No Error" w739 {
        selector: w739 -> [w759 w766]
        tunnel: [w765 w766] -> w748
        tunnel: [w764 w767] -> w747
        tunnel: w738 -> [w755 w767]
        tunnel: w745 -> [w762 _]
        tunnel: w743 -> [w758 _]
        frame No Error {
          n173 = Unbundle By Name(w762) -> ("Amplitude 1"=w761:dbl, "Diffusion Time"=w753:dbl, "Amplitude 2"=w750:dbl, "Translation Time"=w752:dbl, "RMSE"=w760:dbl, "R^2"=w754:dbl)
          n174 = Unbundle By Name(w758) -> ("Amplitude 1"=w757:dbl, "Diffusion Time"=w756:dbl, "Amplitude 2"=w749:dbl, "Translation Time"=w751:dbl)
          n175 = Format Into String(format string=":\nAmplitude 1: %#g ± %#g\nDiffusion Time: %#g ± %#g\nAmplitude 2: %#g ± %#g\nTranslation Time Constant: %#g ± %#g\nMSE: %#g\nR^2: %#g\n", initial string=w755, error in=w759, w761, w757, w753, w756, w750, w749, w752, w751, w760, w754) -> (resulting string=w764:string, error out=w765:errorcluster)
        }
        frame Error {
        }
      }
    }
  }
  n176 = case shown="Error" w5 {
    selector: w5 -> [w769 _]
    tunnel: [w769 w771] -> w4
    tunnel: w3 -> [w768 w773]
    tunnel: "Fit Model" -> [_ w772]
    tunnel: [w768 w770] -> w2
    frame No Error {
    }
    frame Error {
      n177 = Format Into String(format string=": %s Fit Failed!\n", initial string=w773, w772) -> (resulting string=w770:string, error out=w771:errorcluster)  [unwired: 1 in]
    }
  }
  "error out" <- w4
  "Fit Results String" <- w2
